vi "Open.vi"(10 "VI":refnum<vi>) -> ()   [LabVIEW 2025, in "_Shared.lvlib" / "Panel.lvlib"]
uses:
  Panel.lvlib
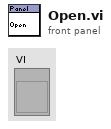
[diagram p1: front panel]
types:
  T1 = enum32{"Invalid", "Standard", "Closed", "Hidden", "Minimized", "Maximized"}
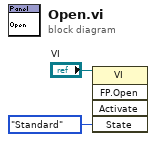
[diagram p0: block diagram]
diagram:
  n1 = invoke class="VI" method="FP.Open"(reference="VI", "State"=T1."Standard") -> ()  [unwired: 3 in, 5 out]
